vi "RT Audio Filter Mathlab Node.vi"() -> ()   [LabVIEW 2022 SP3]
uses:
  <vilib>/FPGAPlugInAG/myRIO-1900/niLvFpga_Open_myRIO-1900.vi
  <vilib>/rvi/interface/common/dynamic/niFpgaDynamicAddResources.vi
  <vilib>/Analysis/3filter.llb/Butterworth Filter (DBL).vi
  <vilib>/Utility/error.llb/Error Cluster From Error Code.vi
  <vilib>/rvi/errors/niLvFpgaAdjustHostInterfaceError.vi
  <vilib>/imath/engines/lvmath2/RunTimeEngine/Managers/WorkSpace/UID Generator.vi
  <vilib>/imath/engines/lvmath2/RunTimeEngine/RunTimeType/NIMS_RunTimeType_From StrictType (excl LVString).vi
  <instcachedir>/0/NIMS_RunTimeType_From StrictType (excl LVString)_FC76839066F94B75B426529F813B8EB7.lvgen/NIMS_RunTimeType_From StrictType (excl LVString)_FC76839066F94B75B426529F813B8EB7_000.vi
  <vilib>/imath/engines/lvmath2/RunTimeEngine/LocalVariableDefStatement/MC_LocalVariableDefStatement_Display.vi
  <vilib>/imath/engines/lvmath2/RunTimeEngine/BuiltInFunctions/iir_butter/NIMS_[2o]_iir_butter(I32,V).vi
  <vilib>/imath/engines/lvmath2/RunTimeEngine/ErrorHandling/NIMS_Error From Error Code.vi
  <vilib>/imath/engines/lvmath2/RunTimeEngine/BuiltInFunctions/filter/NIMS_filter(GV,GV,GV,GV,Str).vi
  <instcachedir>/0/NIMS_filter(GV,GV,GV,GV,Str)_7C5B88D942D8486E8E164CAC1589CA58.lvgen/NIMS_filter(GV,GV,GV,GV,Str)_7C5B88D942D8486E8E164CAC1589CA58_000.vi
  <vilib>/imathl/engines/lvmath/Functions/Error Handling/Create Error.vi
  <vilib>/imath/engines/lvmath2/RunTimeEngine/Managers/SymbolTable/Clear UID.vi
  <vilib>/imath/engines/lvmath2/RunTimeEngine/NodeEndStatement/NIMS_NodeEndStatement_Output.vi
  <instcachedir>/0/NIMS_NodeEndStatement_Output_53EC0D466D134D7ABD903AC30B43404B.lvgen/NIMS_NodeEndStatement_Output_53EC0D466D134D7ABD903AC30B43404B_005.vi
  <vilib>/imath/engines/lvmath2/RunTimeEngine/ErrorHandling/NIMS_Finalize Error.vi
  <vilib>/FPGAPlugInAG/Dynamic/niLvFpga_Close_Dynamic.vi
  <vilib>/rvi/interface/nirviOpenFPGA/nirviOpenFPGA.xnode
  AppData/Local/Temp/45e941dd-0777-4a1f-a0f8-f8ee2228a2c4_tlt4.zip.2c4/tlt4/FPGA Bitfiles/rtaudiofiltermat_FPGATarget_MyCompilation202_r-Juz8rJ+v0.lvbitx
  AppData/Local/Temp/45e941dd-0777-4a1f-a0f8-f8ee2228a2c4_tlt4.zip.2c4/tlt4/FPGA Audio Streaming.vi
  <vilib>/rvi/interface/nirviReadWriteControl/nirviReadWriteControl.xnode
  <vilib>/rvi/interface/nirviCloseFPGA/nirviCloseFPGA.xnode
  <vilib>/Analysis/NI_AALBase.lvlib
  NiFpgaLv.dll
  <vilib>/rvi/interface/Simulation/niFpgaSimulationCallBeginRW.vi
  <vilib>/imath/engines/lvmath2/RunTimeEngine/Managers/SymbolTable/NIMS_WorkSpace.lvlib
panel:
  in  "Gain1":dbl(slide) scale=0.0..10.0
  in  "Gain 5":dbl(slide) scale=0.0..10.0
  in  "Gain4":dbl(slide) scale=0.0..10.0
  in  "Gain3":dbl(slide) scale=0.0..10.0
  in  "Gain2":dbl(slide) scale=0.0..10.0
  out "Model of Computation":string
  in  "Sample Rate (Hz)":dbl=44101.0
  out "Audio Spectrum":dynamicdata(graph)
  in  "Read Rate (Hz)":dbl=5.0
  in  "stop":bool
  # "Audio Equilizer Control"
  # "Application Control"
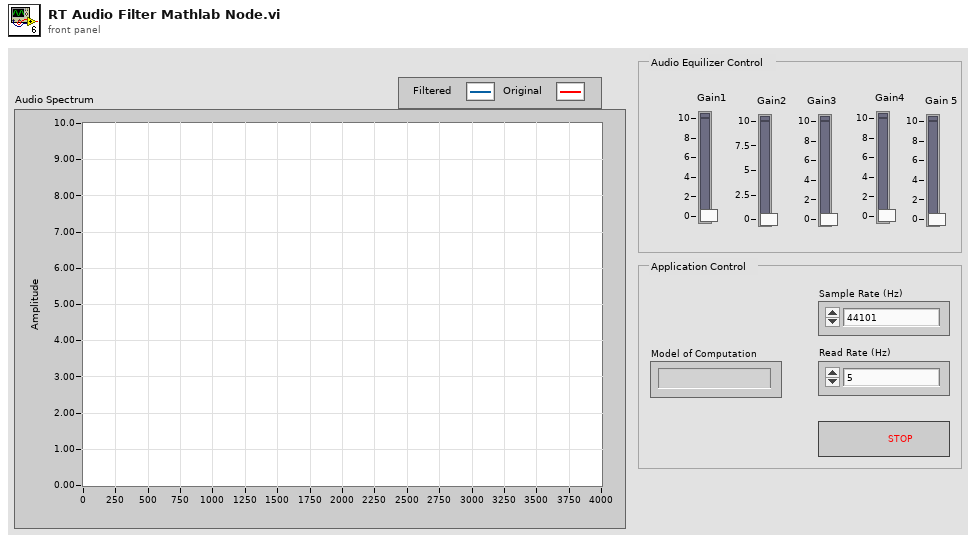
[diagram p1: front panel]
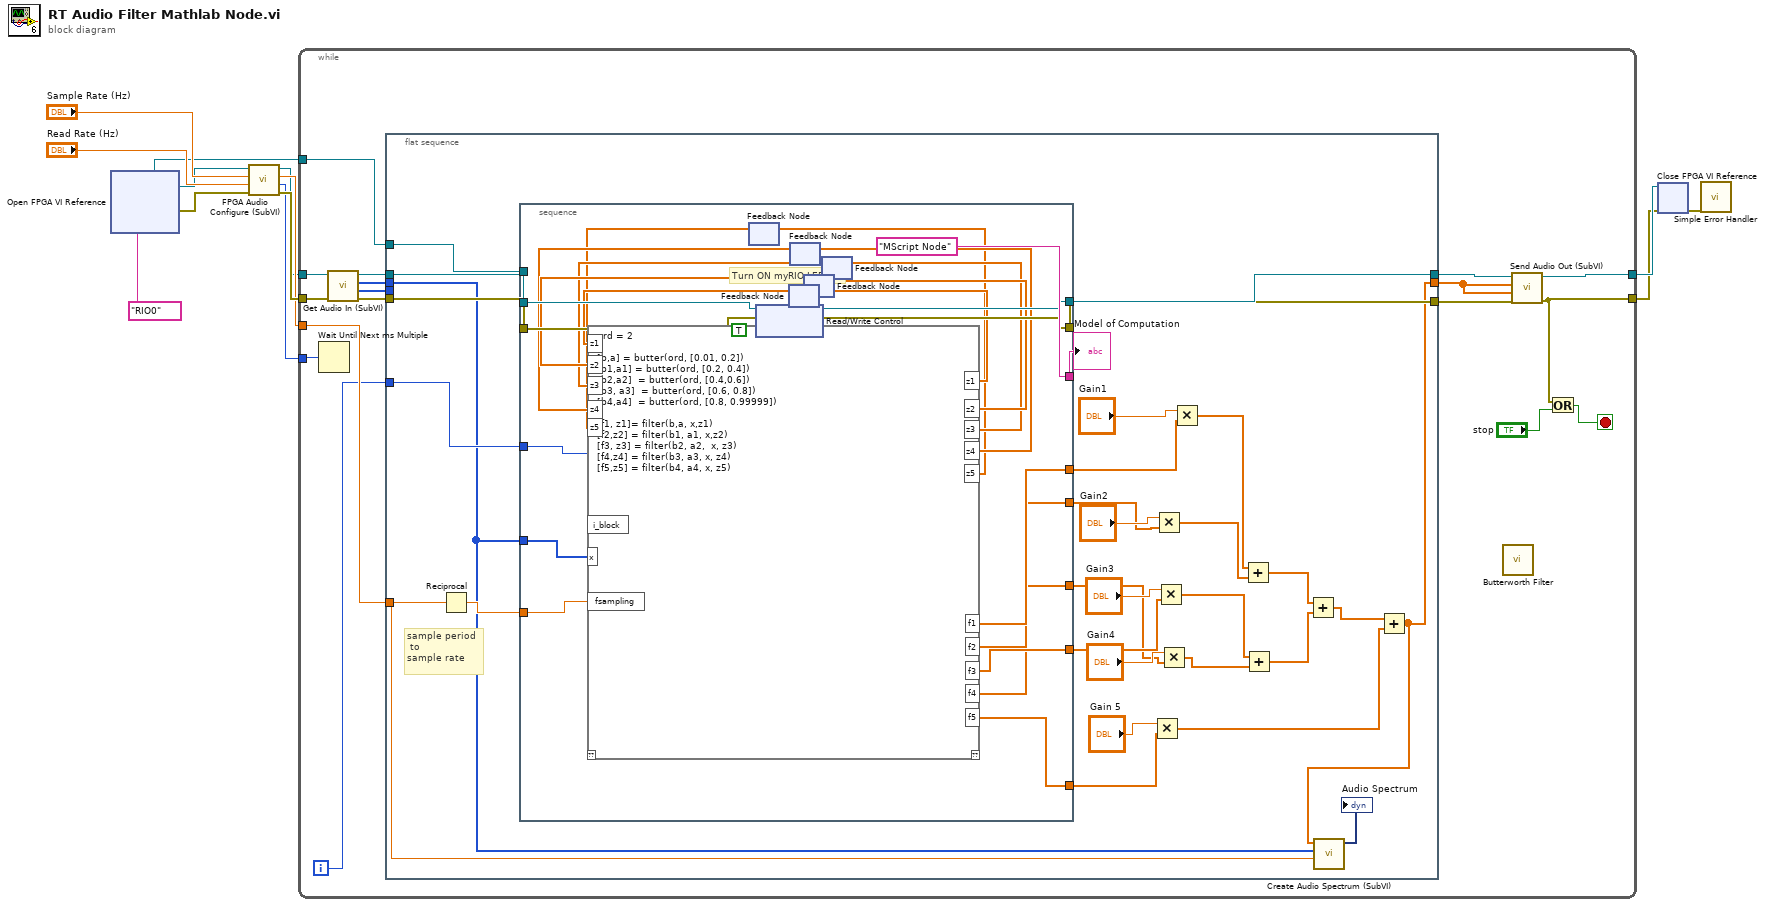
[diagram p0: block diagram]
diagram:
  n1 = xnode "Open FPGA VI Reference"("resource name"=tag "RIO0") -> ("FPGA VI Reference Out"=w1:refnum<k20>, "error out"=w12:errorcluster)  [unwired: 1 in]
  n2 = call "FPGA Audio Configure (SubVI).vi"("error in (no error)"=w12, "Read Rate (Hz)"="Read Rate (Hz)", "Audio Sample Rate (Hz)"="Sample Rate (Hz)", "Refnum in"=w1) -> ("error out"=w8:errorcluster, "Required loop period (ms)"=w3:u32, "Audio dt (ms)"=w5:dbl, "Refnum out"=w2:refnum<k20>)  [unwired: 4 in]
  n3 = while {
    tunnel: w2 -> [w15]
    tunnel: [w26] -> w11
    tunnel: [w22] -> w10
    tunnel: w3 -> [w27]
    tunnel: w8 -> [w28]
    tunnel: w5 -> [w25]
    tunnel: w1 -> [w13]
    i -> [w14]
    stop <- w16 stop-if-true
    n4 = Wait Until Next ms Multiple(millisecond multiple=w27) -> ()  [unwired: 1 out]
    n5 = call "Get Audio In (SubVI).vi"("error in (no error)"=w28, "Refnum in"=w15) -> ("error out"=w20:errorcluster, "Right Audio In"=w17:i16[], "Left Audio In"=w23:i16[], "Refnum out"=w21:refnum<k20>)  [unwired: 6 in]
    n6 = flat-sequence {
      tunnel: w25 -> [w58]
      tunnel: [w30] -> w24
      tunnel: w23 -> [w47]
      tunnel: w21 -> [w55]
      tunnel: w20 -> [w54]
      tunnel: [w53] -> w19
      tunnel: [w52] -> w18
      tunnel: w17 -> [_]
      tunnel: w14 -> [w51]
      tunnel: w13 -> [w32]
      frame #0 {
        # "sample period\n to\nsample rate"
        n7 = Reciprocal(x=w58) -> (1/x=w59:dbl)
        n8 = stacked-sequence {
          tunnel: ["MScript Node" ("Mode")] -> w57
          tunnel: w59 -> [w76]
          tunnel: w47 -> [w77]
          tunnel: w55 -> [w79]
          tunnel: w54 -> [w78]
          tunnel: [w81] -> w53
          tunnel: [w80] -> w52
          tunnel: w51 -> [w75]
          tunnel: [w74] -> w31
          tunnel: [w73] -> w36
          tunnel: [w72] -> w35
          tunnel: [w71] -> w34
          tunnel: [w70] -> w33
          tunnel: w32 -> [_]
          frame #0 {
            # "Turn ON myRIO LEDs"
            n9 = feedback #1() -> (w60:dbl[])  [unwired: 1 in]
            n10 = xnode "Read/Write Control"("FPGA VI Reference In"=w79, "error in"=w78, "LEDs On?"=TRUE) -> ("FPGA VI Reference Out"=w81:refnum<k20>, "error out"=w80:errorcluster)
            n11 = feedback #2() -> (w68:dbl[])  [unwired: 1 in]
            n12 = feedback #3() -> (w62:dbl[])  [unwired: 1 in]
            n13 = feedback #4() -> (w66:dbl[])  [unwired: 1 in]
            n14 = feedback #5() -> (w64:dbl[])  [unwired: 1 in]
            n15 = mathscript code="ord = 2\n\n[b,a] = butter(ord, [0.01, 0.2])\n[b1,a1] = butter(ord, [0.2, 0.4])\n[b2,a2]  = butter(ord, [0.4,0.6])\n[b3, a3]  = butter(ord, [0.6, 0.8])\n[b4,a4]  = butter(ord, [0.8, 0.99999])\n\n[f1, z1]= filter(b,a, x,z1)\n[f2,z2] = filter(b1, a1, x,z2)\n[f3, z3] = filter(b2, a2,  x, z3)\n[f4,z4] = filter(b3, a3, x, z4)\n[f5,z5] = filter(b4, a4, x, z5)"("x"=w77, "fsampling"=w76, "i_block"=w75, "z1"=w68, "z2"=w66, "z3"=w64, "z4"=w62, "z5"=w60) -> ("f1"=w74:dbl[], "f2"=w73:dbl[], "f3"=w72:dbl[], "f4"=w71:dbl[], "f5"=w70:dbl[], "z1"=w69:dbl[], "z2"=w67:dbl[], "z3"=w65:dbl[], "z4"=w63:dbl[], "z5"=w61:dbl[])  [unwired: 1 in, 1 out]
            n16 = feedback-in #1(w61) -> ()
            n17 = feedback-in #2(w69) -> ()
            n18 = feedback-in #3(w63) -> ()
            n19 = feedback-in #4(w67) -> ()
            n20 = feedback-in #5(w65) -> ()
          }
        }
        "Model of Computation" <- w57
        n21 = Multiply(x="Gain 5", y=w33) -> (x*y=w41:dbl[])
        n22 = Multiply(x="Gain2", y=w36) -> (x*y=w45:dbl[])
        n23 = Multiply(x="Gain3", y=w35) -> (x*y=w44:dbl[])
        n24 = Multiply(x="Gain4", y=w34) -> (x*y=w43:dbl[])
        n25 = Multiply(x="Gain1", y=w31) -> (x*y=w39:dbl[])
        n26 = Add(x=w39, y=w45) -> (x+y=w42:dbl[])
        n27 = Add(x=w44, y=w43) -> (x+y=w38:dbl[])
        n28 = Add(x=w42, y=w38) -> (x+y=w40:dbl[])
        n29 = Add(x=w40, y=w41) -> (x+y=w30:dbl[])
        n30 = call "Create Audio Spectrum (SubVI).vi"("Sample Period (ms)"=w58, "Raw Audio"=w47, "Filtered Audio"=w30) -> ("FFT Out"=→"Audio Spectrum":dynamicdata)  [unwired: 8 in]
      }
    }
    n31 = call-poly <vilib>:"Butterworth Filter.vi"() -> ()  [unwired: 8 in, 2 out]
    n32 = call "Send Audio Out (SubVI).vi"("error in (no error)"=w18, "Right Audio Out"=w24, "Left Audio Out"=w24, "Refnum in"=w19) -> ("error out"=w22:errorcluster, "Refnum out"=w26:refnum<k20>)  [unwired: 6 in]
    n33 = Or(x=w22, y="stop") -> (x .or. y?=w16:bool)
  }
  n34 = xnode "Close FPGA VI Reference"("FPGA VI Reference In"=w11, "error in"=w10) -> ("error out"=w4:errorcluster)
  n35 = call <vilib>:"Simple Error Handler.vi"("error in (no error)"=w4) -> ()  [unwired: 4 in, 5 out]
